vi "Virtual FTS.vi"() -> (0 "value":dbl[](array[numeric]))   [LabVIEW 2017]
uses:
  <vilib>/Utility/inputDevices.llb/joystickAcquire.vi
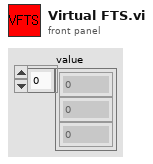
[diagram p1: front panel]
types:
  T1 = cluster{"X axis":i32, "Y axis":i32, "Z axis":i32, "X axis rotation":i32, "Y axis rotation":i32, "Z axis rotation":i32, "U axis":i32, "V axis":i32}
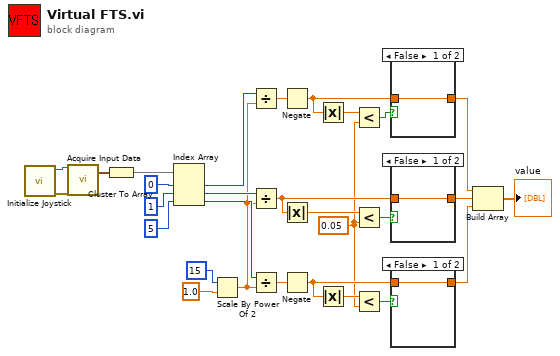
[diagram p0: block diagram]
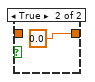
[diagram p2: hidden frame]
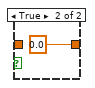
[diagram p3: hidden frame]
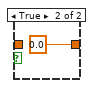
[diagram p4: hidden frame]
diagram:
  w1 = 0.05 ("y")
  n1 = call <vilib>:"Initialize Joystick.vi"() -> ("error out"=w18:errorcluster, "device ID"=w19:refnum<k1>)  [unwired: 10 in]
  n2 = call-poly <vilib>:"Acquire Input Data.vi"("device ID"=w19, "error in (no error)"=w18) -> ("axis info"=w29:T1)  [unwired: 13 in, 4 out]
  n3 = Cluster To Array(cluster=w29) -> (array=w25:i32[])
  n4 = Index Array(array=w25, index #1=0 ("index"), index #2=1 ("index"), index #3=5 ("index")) -> (element #1=w22:i32, element #2=w21:i32, element #3=w20:i32)
  n5 = Scale By Power Of 2(n=i16 15, x=1.0) -> (x*2^n=w13:dbl)
  n6 = Divide(x=w22, y=w13) -> (x/y=w17:dbl)
  n7 = Divide(x=w21, y=w13) -> (x/y=w4:dbl)
  n8 = Divide(x=w20, y=w13) -> (x/y=w2:dbl)
  n9 = Negate(x=w17) -> (-x=w5:dbl)
  n10 = Absolute Value(x=w4) -> (abs(x)=w15:dbl)
  n11 = Negate(x=w2) -> (-x=w3:dbl)
  n12 = Absolute Value(x=w5) -> (abs(x)=w16:dbl)
  n13 = Absolute Value(x=w3) -> (abs(x)=w14:dbl)
  n14 = Less?(x=w16, y=w1) -> (x < y?=w12:bool)
  n15 = Less?(x=w15, y=w1) -> (x < y?=w11:bool)
  n16 = Less?(x=w14, y=w1) -> (x < y?=w10:bool)
  n17 = case shown="False" w12 {
    tunnel: [w30 0.0] -> w9
    tunnel: w5 -> [w30 _]
    frame False {
    }
    frame True {
    }
  }
  n18 = case shown="False" w11 {
    tunnel: [w32 0.0] -> w8
    tunnel: w4 -> [w32 _]
    frame False {
    }
    frame True {
    }
  }
  n19 = case shown="False" w10 {
    tunnel: [w34 0.0] -> w7
    tunnel: w3 -> [w34 _]
    frame False {
    }
    frame True {
    }
  }
  n20 = Build Array(w9, w8, w7) -> (→"value":dbl[])
